vi "Close.vi"(8 "error in":errorcluster, 11 "Thermometer DAQmx RTD Cont CFG in":refnum<class "Thermometer DAQmx RTD Cont CFG.lvclass">) -> (0 "error out":errorcluster, 3 "Thermometer DAQmx RTD Cont CFG out":refnum<class "Thermometer DAQmx RTD Cont CFG.lvclass">)   [LabVIEW 2023, in "Thermometer DAQmx RTD Cont CFG.lvclass"]
uses:
  Thermometer DAQmx RTD Cont CFG.lvclass
  Thermometer DAQmx RTD Cont CFG.lvclass/Thermometer DAQmx RTD Cont CFG.ctl
  DAQmx/DAQmx Base CFG/DAQmx Base CFG.lvclass
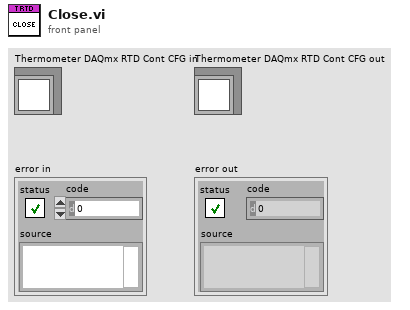
[diagram p1: front panel]
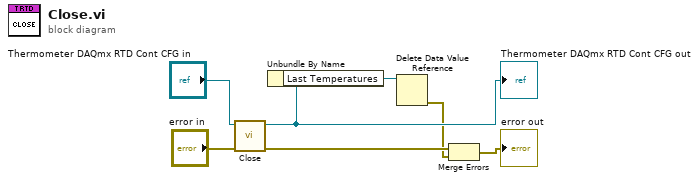
[diagram p0: block diagram]
diagram:
  n1 = call-parent "Close.vi"("error in"="error in", "DAQmx Base CFG in"="Thermometer DAQmx RTD Cont CFG in") -> ("error out"=w7:errorcluster, "DAQmx Base CFG out"=w4:refnum<class "Thermometer DAQmx RTD Cont CFG.lvclass">)  [unwired: 8 in]
  "Thermometer DAQmx RTD Cont CFG out" <- w4
  n2 = Unbundle By Name(w4) -> ("Last Temperatures"=w3:refnum<data-value>)
  n3 = Delete Data Value Reference(data value reference=w3) -> (error out=w1:errorcluster)  [unwired: 1 in, 1 out]
  n4 = Merge Errors(w7, w1) -> (→"error out":errorcluster)
